vi "Send Request.vi"(8 "error in (no error)":errorcluster, 11 "HTTP Session in":refnum<class "Session.lvclass">) -> (0 "error out":errorcluster, 1 "Response body":string, 2 "Response headers":string, 3 "HTTP Session out":refnum<class "Session.lvclass">)   [LabVIEW 2015, in "NI_Azure_Core.lvlib" / "Session.lvclass"]
uses:
  Session.lvclass
  Session.lvclass/Session.ctl
  Read HTTP Verb.vi
  Read Request body.vi
  Read HTTP Session.vi
  Read Storage Account URI.vi
  Read Content Length.vi
  <vilib>/httpClient/PUTBuffer.vi
  <vilib>/httpClient/POSTBuffer.vi
  <vilib>/httpClient/LabVIEWHTTPClient.lvlib
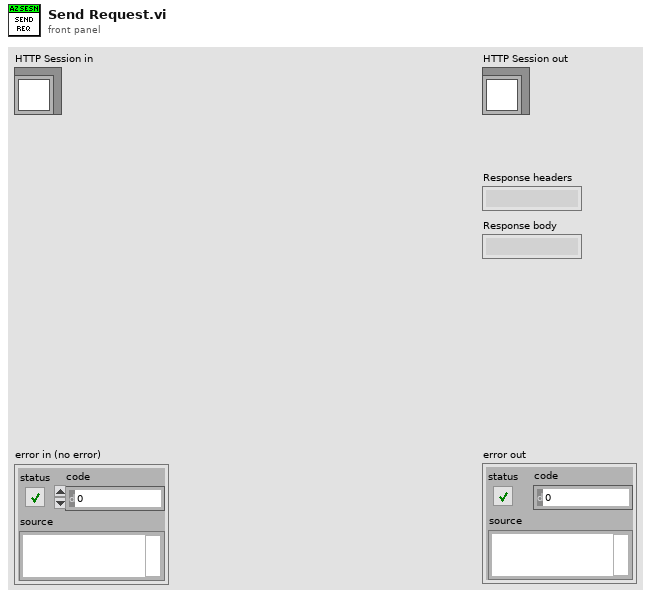
[diagram p1: front panel]
types:
  T1 = typedef "LabVIEWHTTPClient.lvlib/ClientHandle.ctl" = refnum<k1>
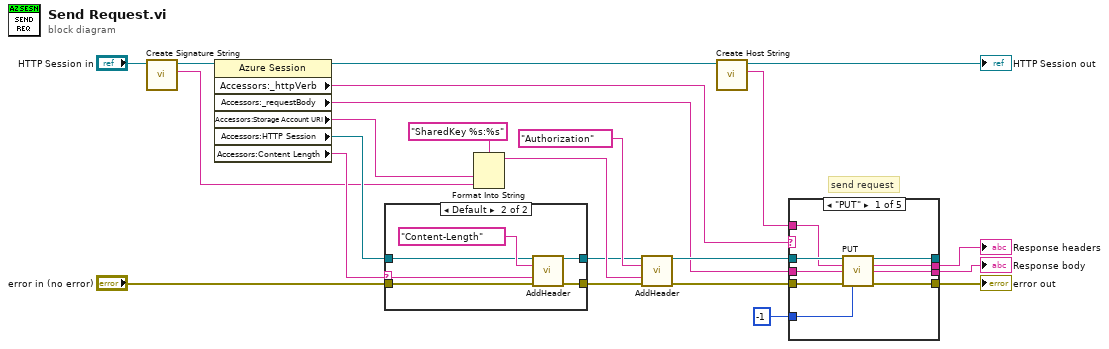
[diagram p0: block diagram]
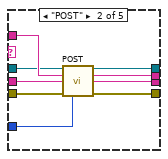
[diagram p3: hidden frame]
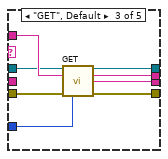
[diagram p4: hidden frame]
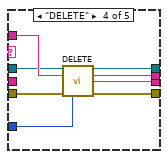
[diagram p5: hidden frame]
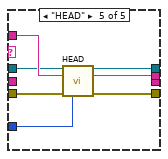
[diagram p6: hidden frame]
diagram:
  # "send request"
  n1 = call "Create Signature String.vi"("HTTP Session in"="HTTP Session in") -> ("Encoded signature"=w2:string, "HTTP Session out"=w3:refnum<class "Session.lvclass">)  [unwired: 8 in]
  n2 = property class="Azure Session"(reference=w3) -> (reference out=w6:refnum<class "Session.lvclass">, "Accessors:_httpVerb"=w8:string, "Accessors:_requestBody"=w9:string, "Accessors:Storage Account URI"=w10:string, "Accessors:HTTP Session"=w11:T1, "Accessors:Content Length"=w12:string)  [unwired: 1 in, 1 out]
  n3 = case shown="Default" w12 {
    selector: w12 -> [_ w31]
    tunnel: [w25 w29] -> w15
    tunnel: "error in (no error)" -> [w25 w28]
    tunnel: w11 -> [w24 w27]
    tunnel: [w24 w26] -> w14
    frame "0" {
    }
    frame Default {
      n4 = call <vilib>:"AddHeader.vi"("client handle"=w27, "header"="Content-Length", "value"=w31, "error in (no error)"=w28) -> ("client handle out"=w26:T1, "error out"=w29:errorcluster)  [unwired: 10 in]
    }
  }
  n5 = Format Into String(format string="SharedKey %s:%s", w10, w2) -> (resulting string=w17:string)  [unwired: 2 in, 1 out]
  n6 = call <vilib>:"AddHeader.vi"("client handle"=w14, "header"="Authorization", "value"=w17, "error in (no error)"=w15) -> ("client handle out"=w19:T1, "error out"=w23:errorcluster)  [unwired: 10 in]
  n7 = call "Create Host String.vi"("HTTP Session in"=w6) -> ("Host String"=w7:string, "HTTP Session out"=→"HTTP Session out":refnum<class "Session.lvclass">)  [unwired: 9 in]
  n8 = case shown="\"PUT\"" w8 {
    tunnel: [w35 w49 w56 w60 _] -> w20
    tunnel: [w34 w48 w57 w59 w72] -> w21
    tunnel: w7 -> [w39 w47 w53 w63 w70]
    tunnel: w19 -> [w40 w46 w52 w62 w68]
    tunnel: w9 -> [w38 w45 _ _ _]
    tunnel: w23 -> [w37 w44 w54 w64 w69]
    tunnel: [w36 w43 w55 w65 w71] -> w13
    tunnel: [w33 w42 w51 w61 w67] -> _
    tunnel: -1 ("timeout (10000)") -> [w32 w41 w50 w58 w66]
    frame "PUT" {
      n9 = call-poly <vilib>:"PUT.vi"("client handle"=w40, "url"=w39, "buffer"=w38, "error in (no error)"=w37, "timeout (10000)"=w32) -> ("client handle out"=w33:T1, "headers"=w34:string, "body"=w35:string, "error out"=w36:errorcluster)  [unwired: 7 in]
    }
    frame "POST" {
      n10 = call-poly <vilib>:"POST.vi"("client handle"=w46, "url"=w47, "buffer"=w45, "error in (no error)"=w44, "timeout (10000)"=w41) -> ("client handle out"=w42:T1, "headers"=w48:string, "body"=w49:string, "error out"=w43:errorcluster)  [unwired: 7 in]
    }
    frame "GET", Default {
      n11 = call <vilib>:"GET.vi"("client handle"=w52, "url"=w53, "error in (no error)"=w54, "timeout (10000)"=w50) -> ("client handle out"=w51:T1, "headers"=w57:string, "body"=w56:string, "error out"=w55:errorcluster)  [unwired: 8 in]
    }
    frame "DELETE" {
      n12 = call <vilib>:"DELETE.vi"("client handle"=w62, "url"=w63, "error in (no error)"=w64, "timeout (10000)"=w58) -> ("client handle out"=w61:T1, "headers"=w59:string, "body"=w60:string, "error out"=w65:errorcluster)  [unwired: 8 in]
    }
    frame "HEAD" {
      n13 = call <vilib>:"HEAD.vi"("client handle"=w68, "url"=w70, "error in (no error)"=w69, "timeout (10000)"=w66) -> ("client handle out"=w67:T1, "headers"=w72:string, "error out"=w71:errorcluster)  [unwired: 9 in]
    }
  }
  "Response headers" <- w21
  "Response body" <- w20
  "error out" <- w13
